vi "readScanCommand.vi"(8 "error in":errorcluster, 11 "FPGA VI Reference In":refnum<k20>) -> (0 "error out":errorcluster, 2 "scan command":T1, 3 "FPGA VI Reference Out":refnum<k20>)   [LabVIEW 2010]
uses:
  <vilib>/rvi/interface/nirviMethod/nirviMethod.xnode
  <vilib>/rvi/interface/common/niFpgaNodeNameForErrorReporting.ctl
  <vilib>/rvi/errors/niLvFpgaWhatHappensToTopLevelVI.ctl
  <vilib>/Utility/error.llb/Error Cluster From Error Code.vi
  <vilib>/rvi/errors/niLvFpgaAdjustHostInterfaceError.vi
  NiFpgaLv.dll
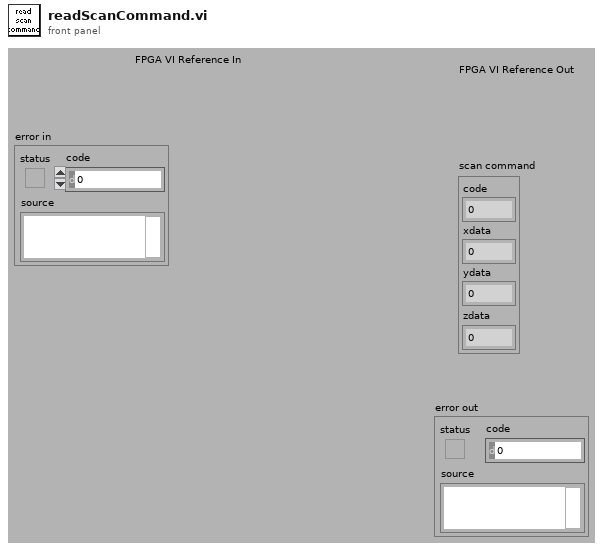
[diagram p1: front panel]
types:
  T1 = cluster{"code":i32, "xdata":i32, "ydata":i32, "zdata":i32}
  T2 = cluster{"Data[0]":i32, "Data[1]":i32, "Data[2]":i32, "Data[3]":i32}
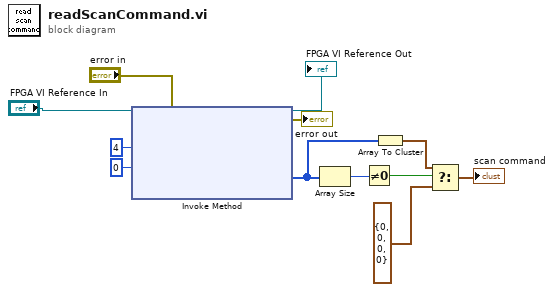
[diagram p0: block diagram]
diagram:
  n1 = xnode "Invoke Method"("FPGA VI Reference In"="FPGA VI Reference In", "error in"="error in", "Number of Elements"=u32 4, "Timeout (ms)"=0) -> ("FPGA VI Reference Out"=→"FPGA VI Reference Out":refnum<k20>, "error out"=→"error out":errorcluster, "Data"=w5:i32[])  [unwired: 1 out]
  n2 = Array Size(array=w5) -> (size(s)=w6:i32)
  n3 = Not Equal To 0?(x=w6) -> (x != 0?=w4:bool)
  n4 = Array To Cluster(array=w5) -> (cluster=w3:T2)
  n5 = Select(t=w3, s=w4, f=T2 {"Data[0]"=0, "Data[1]"=0, "Data[2]"=0, "Data[3]"=0}) -> (s? t:f=→"scan command":T2)
